vi "PlateReaderV2.vi"() -> ()   [LabVIEW 2014]
uses:
  ReadSpecifications.ctl
  TimingProfile.ctl
  PlateReaderState.ctl
  ColumnData.ctl
  RPMUpdateData.ctl
  MasterCluster.ctl
  EventHandleCommandCompletedData.ctl
  EventHandleErrorReportData.ctl
  PlateReaderGlobal.vi
  <vilib>/Instr/_visa.llb/VISA Configure Serial Port (Instr).vi
  C:/Program Files (x86)/Molecular Devices/SoftMax Pro 6.5.1 Automation SDK/SoftMaxPro.AutomationClient.dll
  Program Files (x86)/Molecular Devices/SoftMax Pro 6.5.1 Automation SDK/SoftMaxPro.AutomationClient.dll
  <vilib>/regexp/Match Regular Expression.xnode
panel:
  in  "Arduino COM Port":refnum<visa-resource-name>
  in  "Send Spoof Speed":bool
  in  "Spoof Speed (RPM)":dbl
  in  "Clear Mark Read":bool
  in  "Mark Read Stop":bool
  in  "Mark Read Start":bool
  out "Speed (RPM)":dbl
  out "Last RPM Update Time":timestamp format="%<%H:%M:%S\n%x>T"
  out "Experiment Start Time":timestamp format="%<%H:%M:%S\n%x>T"
  out "Read Count":u64
  out "Loop Iteration":i32
  out "Active Column":u64
  out "SpectraMax M5e Hardware State":string
  out "Last Column Data":T1 {"Column Mark Read Stop Time" format="%<%H:%M:%S%3u\n%x>T"; "Column Mark Read Start Time" format="%<%H:%M:%S%3u\n%x>T"; "Column Busy Stop Time" format="%<%H:%M:%S%3u\n%x>T"; "Column Busy Start Time" format="%<%H:%M:%S%3u\n%x>T"; "Column Read Start Time" format="%<%H:%M:%S%3u\n%x>T"; "Col Read Times" format="%<%H:%M:%S%3u\n%x>T"}
  out "Speed (RPM)":dbl(knob) scale=0.0..15.0
  out "Last Measured Absorbances":string[][](array[string])
  out "Position (deg)":dbl(knob) scale=0.0..360.0
  out "Message Log":string
  in  "Stop":bool
  out "LabVIEW Software State":T2
  out "SMP Return String":string
  in  "Read Specifications":T3={"Read Period (min)"=0.0, "Experiment Duration (min)"=3600.0, "Number of Columns"=12, "Apex Deviance (deg)"=90.0, "Log File Name"="Log", "Number of Wavelengths"=1, "Timing Profile"=enum."No Timing", "Column Switch Delay"=0.0, "Column Repeat Delay"=0.0, "Audible Read Delay"=0.0, "Audible Read Interval"=0.0, "SMP Protocol Path"=path "", "Upper Busy Delay Limit"=inf, "Lower Busy Delay Limit"=-inf, "Upper Busy Interval Limit"=inf, "Lower Busy Interval Limit"=-inf, "Number of Rows"=0, "Plate Reader COM Port"=""}
  in  "Start":bool
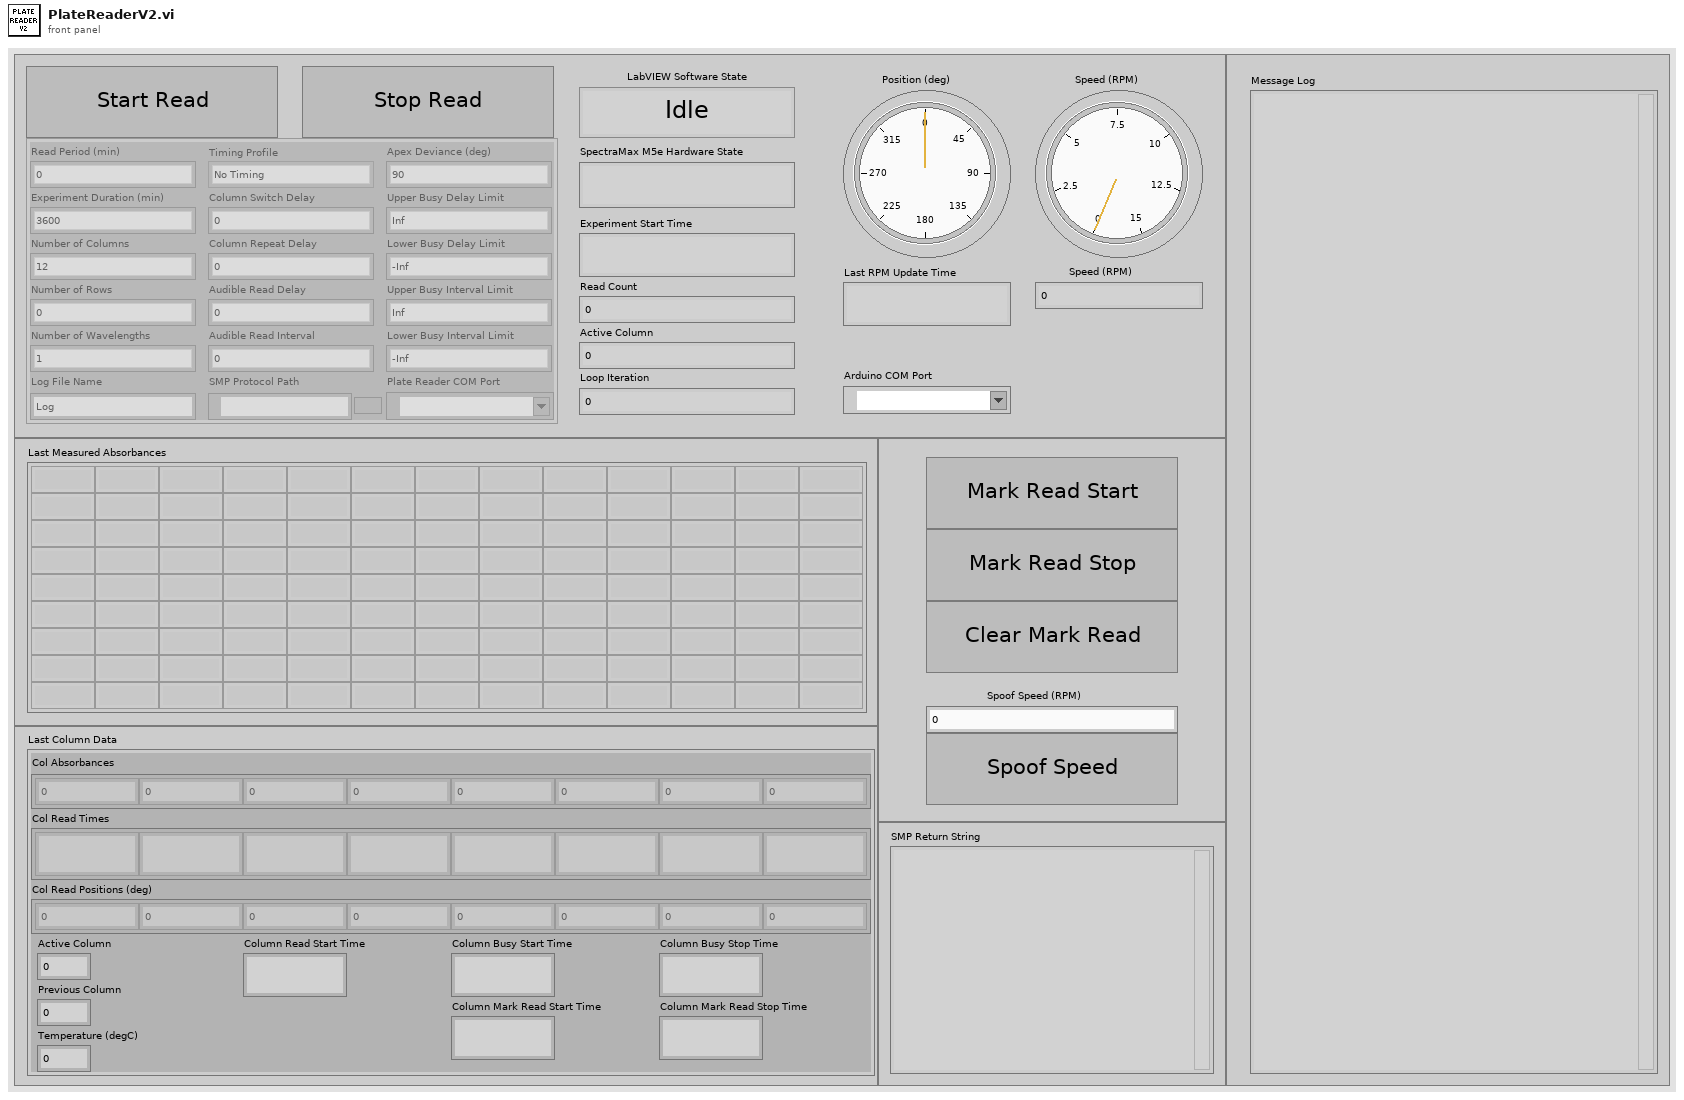
[diagram p1: front panel]
types:
  T1 = typedef "ColumnData.ctl" = cluster{"Col Absorbances":dbl[], "Col Read Times":timestamp[], "Col Read Positions (deg)":dbl[], "Temperature (degC)":dbl, "Active Column":u64, "Previous Column":u64, "Column Read Start Time":timestamp, "Column Busy Start Time":timestamp, "Column Busy Stop Time":timestamp, "Column Mark Read Start Time":timestamp, "Column Mark Read Stop Time":timestamp}
  T2 = typedef "PlateReaderState.ctl" = enum16{"Idle", "Run", "Wait", "Read", "Init", "Exit", "Stop"}
  T3 = typedef "ReadSpecifications.ctl" = cluster{"Read Period (min)":dbl, "Experiment Duration (min)":dbl, "Number of Columns":u64, "Apex Deviance (deg)":dbl, "Log File Name":string, "Number of Wavelengths":u64, "Timing Profile":T4, "Column Switch Delay":dbl, "Column Repeat Delay":dbl, "Audible Read Delay":dbl, "Audible Read Interval":dbl, "SMP Protocol Path":path, "Upper Busy Delay Limit":dbl, "Lower Busy Delay Limit":dbl, "Upper Busy Interval Limit":dbl, "Lower Busy Interval Limit":dbl, "Number of Rows":u64, "Plate Reader COM Port":refnum<visa-resource-name>}
  T4 = typedef "TimingProfile.ctl" = enum16{"No Timing", "24-Well Fluorescence", "48-Well Fluorescence", "96-Well Fluorescence", "96-Well Absorbance", "Custom Timing"}
  T5 = typedef "MasterCluster.ctl" = cluster{"Plate Reader State":T2, "SMPAutomationClientRef":refnum<k24>, "CommandCompleted Refnum":refnum<k27>, "InstrumentStatusChanged Refnum":refnum<k27>, "ErrorReport Refnum":refnum<k27>, "Read Start Time":timestamp, "Read Count":u64, "Active Column":u64, "Raw Result":string, "GetDataCopy CMD Queue ID":i32, "Error Log":string, "Column Data":T1, "Grid":dbl[][], "Column Read Start Time":timestamp, "Previous Column":u64, "Raw Log File Refnum":refnum<file>, "Read Specifications":T3, "Plate Reader Crash State":T2, "Consecutive Missed Reads":u64, "Excel File Refnum":refnum<file>}
  T6 = typedef "RPMUpdateData.ctl" = cluster{"RPM":dbl, "Last RPM Update":timestamp, "Last Position (deg)":dbl}
  T7 = typedef "EventHandleInstrumentStatusChangedData.ctl" = cluster{"Event Common Data":cluster{"Event Source":i32, "Event Type":u32, "Time Stamp":u32}, "Status":string}
  T8 = enum8{"Enabled", "Disabled", "Disabled and Grayed Out"}
  T9 = typedef "EventHandleErrorReportData.ctl" = cluster{"Event Common Data":cluster{"Event Source":i32, "Event Type":u32, "Time Stamp":u32}, "Error":string, "Command ID":i32}
  T10 = typedef "EventHandleCommandCompletedData.ctl" = cluster{"Event Common Data":cluster{"Event Source":i32, "Event Type":u32, "Time Stamp":u32}, "CommandID":i32, "DoubleResult":dbl, "IntResult":i32, "QueueEmpty":bool, "QueueID":i32, "StringResult":string}
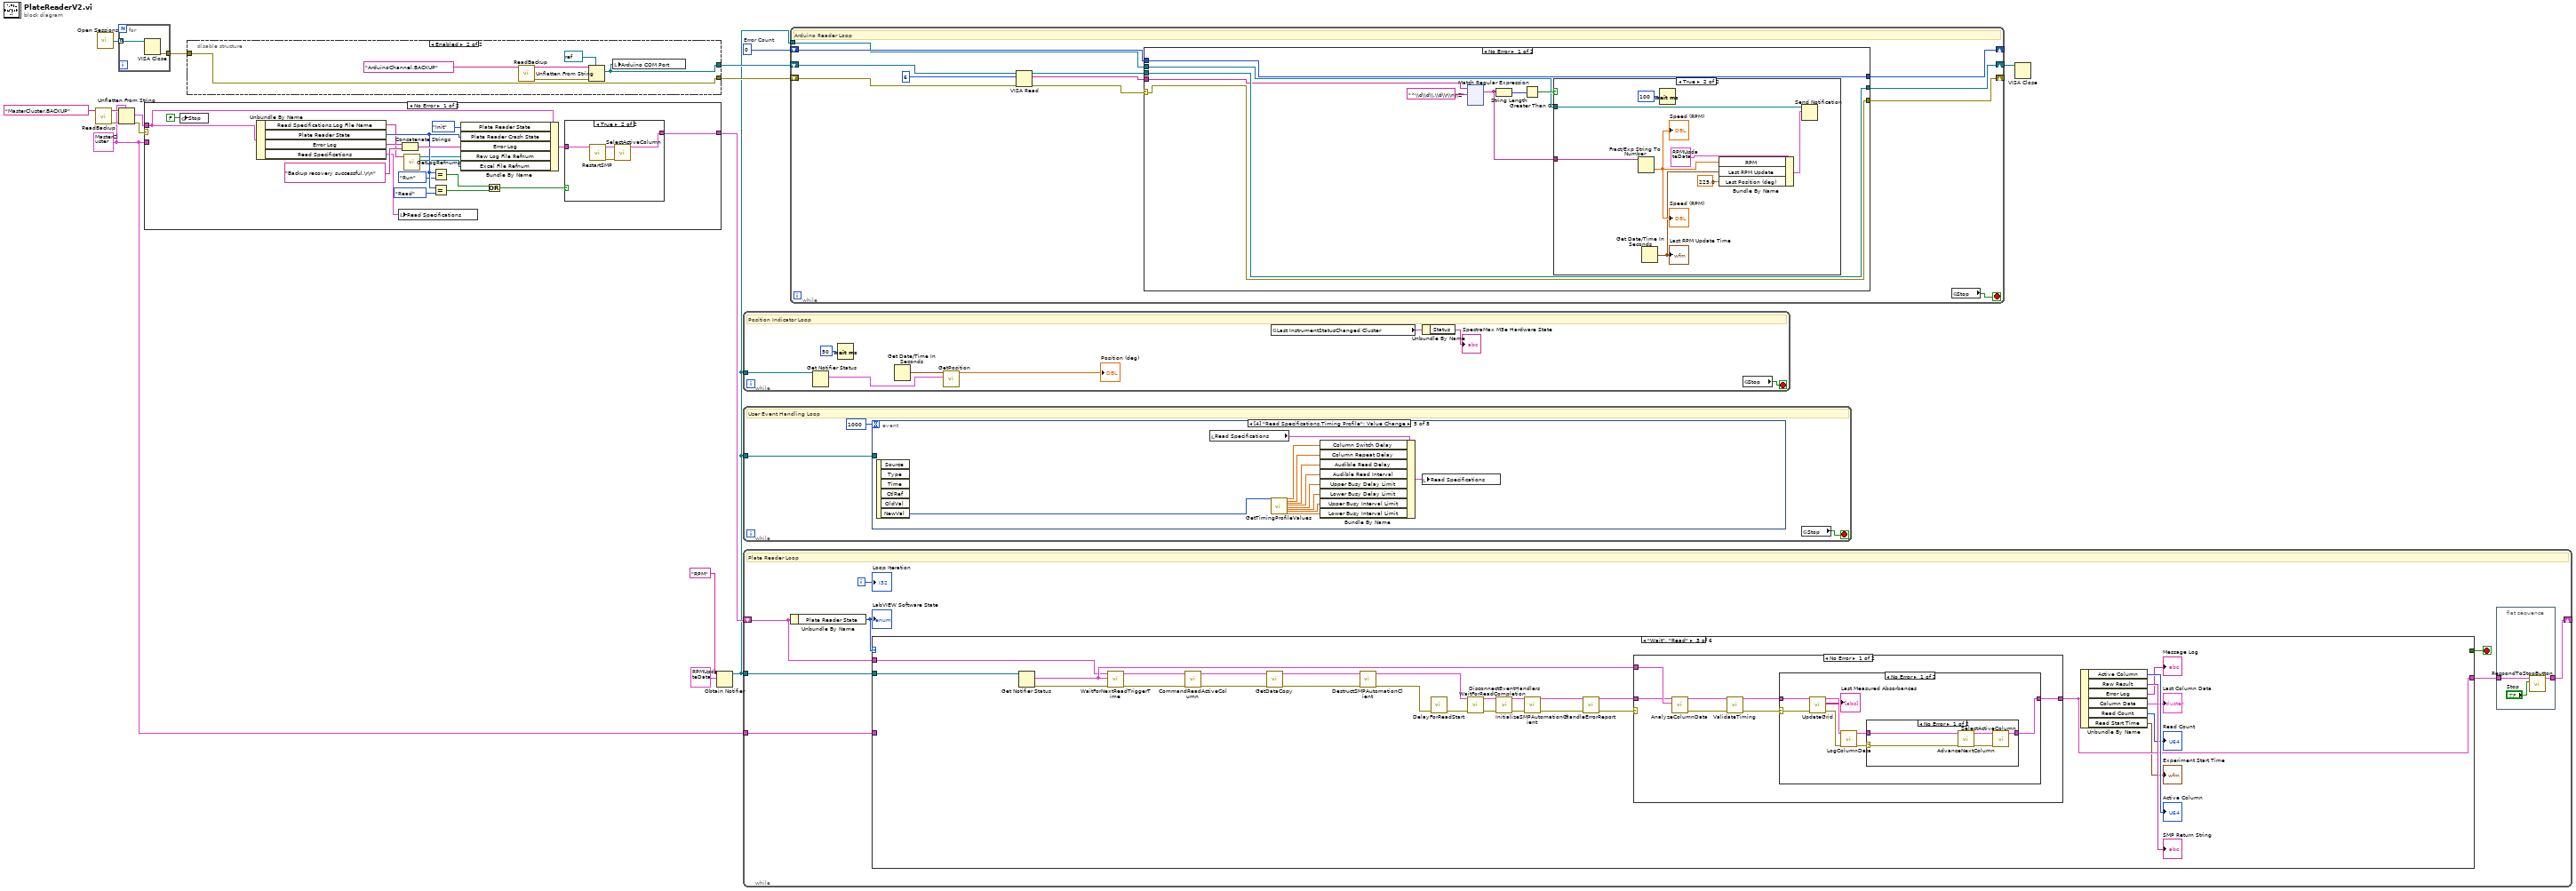
[diagram p0: block diagram]
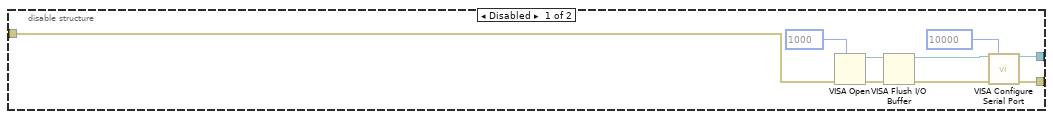
[diagram p2: hidden frame]
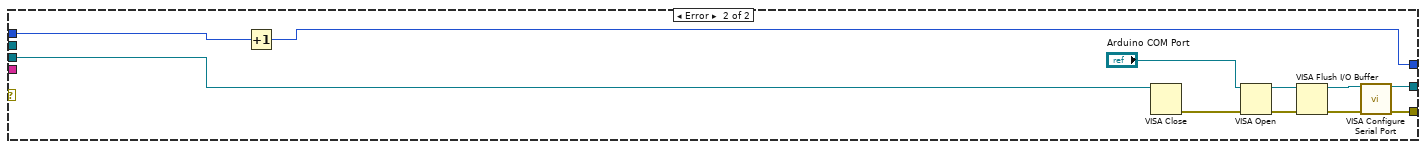
[diagram p4: hidden frame]
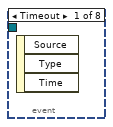
[diagram p5: hidden frame]
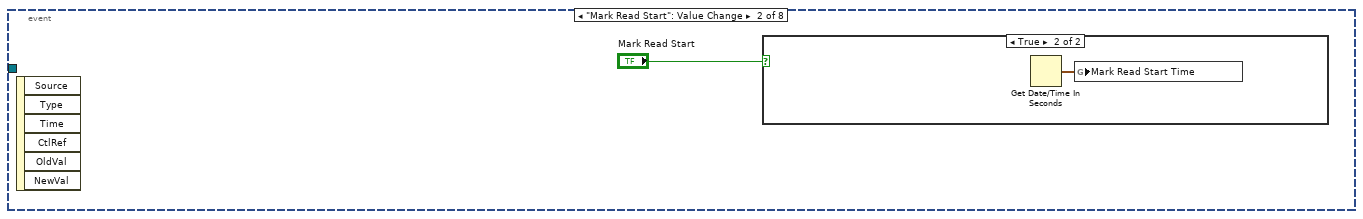
[diagram p6: hidden frame]
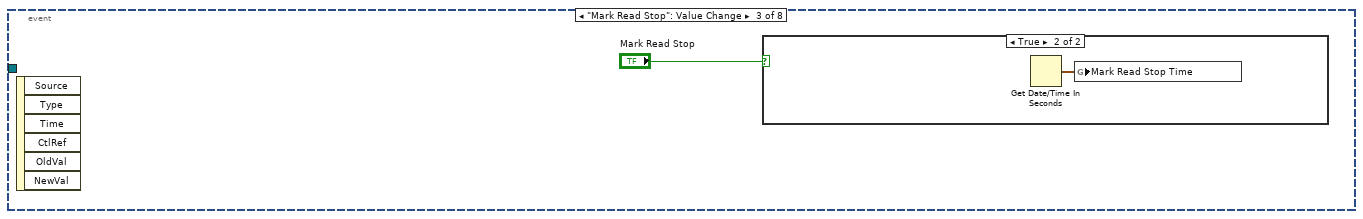
[diagram p8: hidden frame]
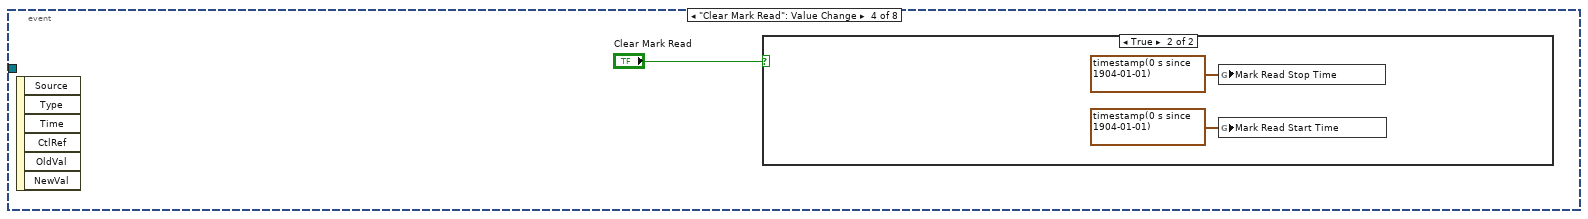
[diagram p10: hidden frame]
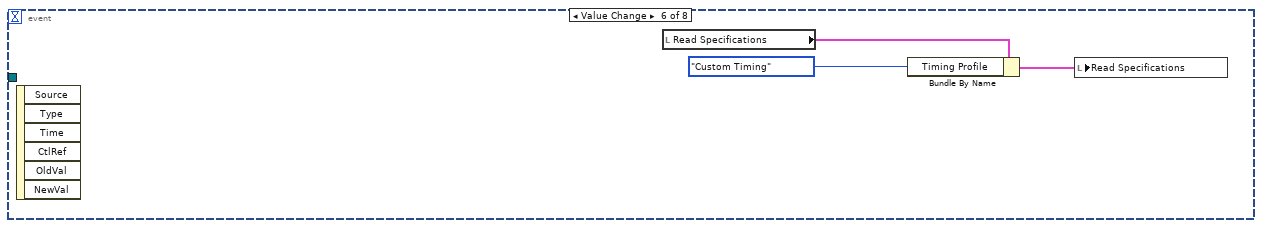
[diagram p12: hidden frame]
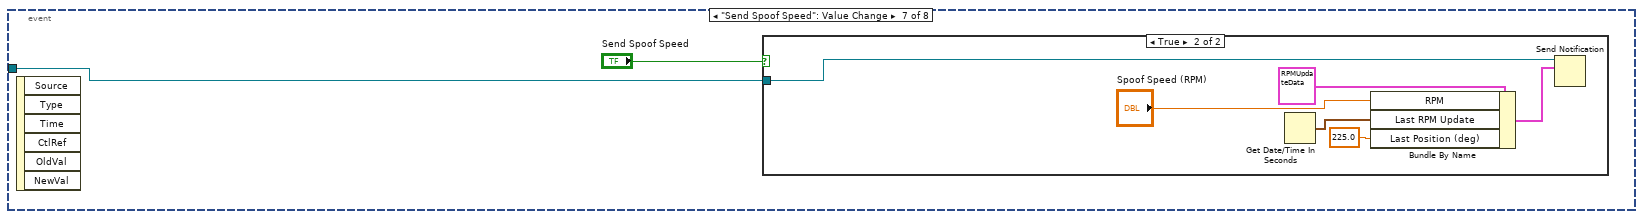
[diagram p13: hidden frame]
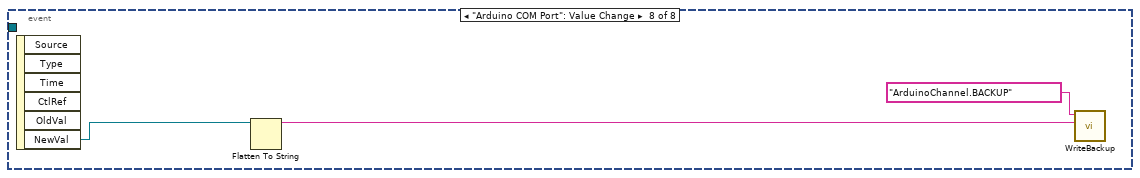
[diagram p15: hidden frame]
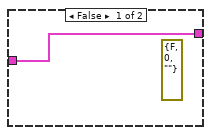
[diagram p16: hidden frame]
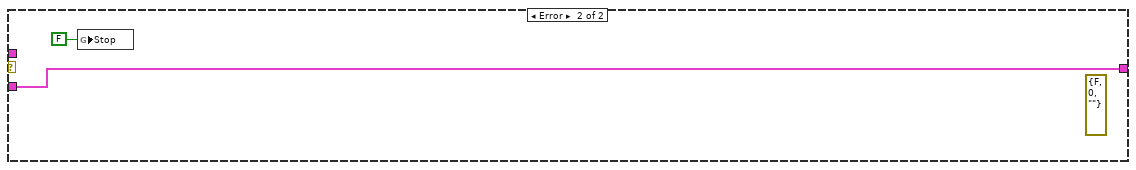
[diagram p17: hidden frame]
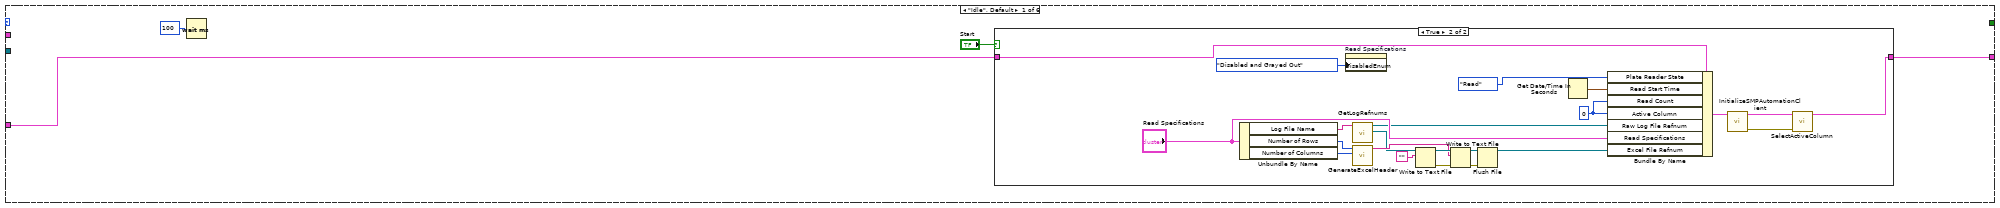
[diagram p18: hidden frame]
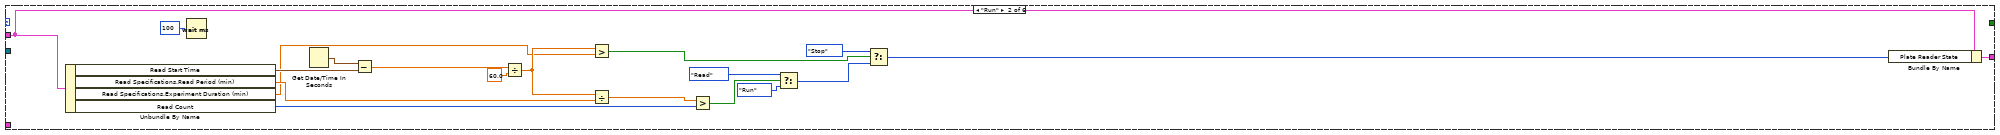
[diagram p20: hidden frame]
diagram:
  w8 = 0  # Error Count
  w1 = T5 {"Plate Reader State"=enum."Init", "SMPAutomationClientRef"=refnum, "CommandCompleted Refnum"=refnum, "InstrumentStatusChanged Refnum"=refnum, "ErrorReport Refnum"=refnum, "Read Start Time"=timestamp(0 s since 1904-01-01), "Read Count"=0, "Active Column"=0, "Raw Result"="", "GetDataCopy CMD Queue ID"=0, "Error Log"="", "Column Data"={"Col Absorbances"=[], "Col Read Times"=[], "Col Read Positions (deg)"=[], "Temperature (degC)"=0.0, "Active Column"=0, "Previous Column"=0, "Column Read Start Time"=timestamp(0 s since 1904-01-01), "Column Busy Start Time"=timestamp(0 s since 1904-01-01), "Column Busy Stop Time"=timestamp(0 s since 1904-01-01), "Column Mark Read Start Time"=timestamp(0 s since 1904-01-01), "Column Mark Read Stop Time"=timestamp(0 s since 1904-01-01)}, "Grid"=[[nan, nan, nan, nan, nan, nan, nan, nan, nan, nan, nan, nan], [nan, nan, nan, nan, nan, nan, nan, nan, nan, nan, nan, nan], [nan, nan, nan, nan, nan, nan, nan, nan, nan, nan, nan, nan], [nan, nan, nan, nan, nan, nan, nan, nan, nan, nan, nan, nan], [nan, nan, nan, nan, nan, nan, nan, nan, nan, nan, nan, nan], [nan, nan, nan, nan, nan, nan, nan, nan, nan, nan, nan, nan], [nan, nan, nan, nan, nan, nan, nan, nan, nan, nan, nan, nan], [nan, nan, nan, nan, nan, nan, nan, nan, nan, nan, nan, nan]], "Column Read Start Time"=timestamp(0 s since 1904-01-01), "Previous Column"=0, "Raw Log File Refnum"=refnum, "Read Specifications"={"Read Period (min)"=0.0, "Experiment Duration (min)"=0.0, "Number of Columns"=0, "Apex Deviance (deg)"=0.0, "Log File Name"="", "Number of Wavelengths"=0, "Timing Profile"=enum."No Timing", "Column Switch Delay"=0.0, "Column Repeat Delay"=0.0, "Audible Read Delay"=0.0, "Audible Read Interval"=0.0, "SMP Protocol Path"=path "", "Upper Busy Delay Limit"=inf, "Lower Busy Delay Limit"=-inf, "Upper Busy Interval Limit"=inf, "Lower Busy Interval Limit"=-inf, "Number of Rows"=0, "Plate Reader COM Port"=""}, "Plate Reader Crash State"=enum."Idle", "Consecutive Missed Reads"=0, "Excel File Refnum"=refnum} ("MasterCluster")
  n1 = call "ReadBackup.vi"("Backup Name"="MasterCluster.BACKUP" ("name or relative path")) -> ("error out"=w2:errorcluster, "Backup Data"=w4:string)  [unwired: 9 in]
  n2 = call <vilib>:"Open Sessions.vi"() -> ("Array of Refnums"=w10:refnum<visa-resource-name>[])  [unwired: 2 in]
  n3 = for {
    tunnel: w10 -> [w18] mode=indexing
    tunnel: [w17] -> w9
    n4 = VISA Close(VISA resource name=w18) -> (error out=w17:errorcluster)  [unwired: 1 in]
  }
  n5 = Unflatten From String(type=w1, binary string=w4, error in (no error)=w2) -> (value=w12:T5, error out=w14:errorcluster)  [unwired: 2 in, 1 out]
  n6 = case shown="No Error" w14 {
    tunnel: [w27 w43] -> w13
    tunnel: w1 -> [_ w43]
    tunnel: w12 -> [w30 _]
    frame No Error {
      n7 = global write "PlateReaderGlobal.vi" "Stop"(FALSE ("Stop")) -> ()
      n8 = Unbundle By Name(w30) -> ("Read Specifications.Log File Name"=w21:string, "Plate Reader State"=w26:T2, "Error Log"=w35:string, "Read Specifications"=w31:T3)
      n9 = local write "Read Specifications"(w31) -> ()
      n10 = Concatenate Strings(w35, "Backup recovery successful.\r\n" ("string")) -> (w33:string)
      n11 = call "GetLogRefnums.vi"("Log File Name"=w21) -> ("Excel Log Refnum"=w19:refnum<file>, "Raw Log Refnum"=w20:refnum<file>)  [unwired: 9 in]
      n12 = Equal?(x=w26, y=PlateReaderState."Run") -> (x = y?=w24:bool)
      n13 = Equal?(x=w26, y=PlateReaderState."Read") -> (x = y?=w23:bool)
      n14 = Bundle By Name(cluster=w30, "Plate Reader State"=PlateReaderState."Init", "Plate Reader Crash State"=w26, "Error Log"=w33, "Raw Log File Refnum"=w20, "Excel File Refnum"=w19) -> (w28:T5)
      n15 = Or(x=w24, y=w23) -> (x .or. y?=w22:bool)
      n16 = case shown="True" w22 {
        tunnel: w28 -> [w37 w40]
        tunnel: [w37 w41] -> w27
        frame False {
          (unwired) errorcluster {"status"=FALSE, "code"=0, "source"=""} ("Error Out")
        }
        frame True {
          n17 = call "RestartSMP.vi"("MasterCluster In"=w40) -> ("Error Out"=w38:errorcluster, "MasterCluster Out"=w39:T5)  [unwired: 9 in]
          n18 = call "SelectActiveColumn.vi"("Error In"=w38, "MasterCluster In"=w39) -> ("MasterCluster Out"=w41:T5)  [unwired: 8 in, 1 out]
        }
      }
    }
    frame Error {
      (unwired) errorcluster {"status"=FALSE, "code"=0, "source"=""} ("Error Out")
      n19 = global write "PlateReaderGlobal.vi" "Stop"(FALSE ("Stop")) -> ()
    }
  }
  n20 = disable-structure shown="Enabled" {
    disable-tunnel: w9 -> [w50 w58]
    disable-tunnel: [w47 w53] -> w7
    disable-tunnel: [w46 w58] -> w6
    frame Disabled {
      n21 = VISA Open(timeout (0)=u32 1000 ("VISA Open timeout (0)"), error in (no error)=w50) -> (VISA resource name=w51:refnum<visa-resource-name>, error out=w49:errorcluster)  [unwired: 3 in]
      n22 = VISA Flush I/O Buffer(VISA resource name=w51, error in (no error)=w49) -> (VISA resource name out=w52:refnum<visa-resource-name>, error out=w48:errorcluster)  [unwired: 1 in]
      n23 = call-poly "VISA Configure Serial Port"("VISA resource name"=w52, "timeout (10sec)"=u32 10000, "error in (no error)"=w48) -> ("VISA resource name out"=w47:refnum<visa-resource-name>, "error out"=w46:errorcluster)  [unwired: 11 in]
    }
    frame Enabled {
      n24 = call "ReadBackup.vi"("Backup Name"="ArduinoChannel.BACKUP" ("name or relative path")) -> ("error out"=w57:errorcluster, "Backup Data"=w55:string)  [unwired: 9 in]
      n25 = Unflatten From String(type=refnum<visa-resource-name> refnum ("VISA resource name out"), binary string=w55, error in (no error)=w57) -> (value=w53:refnum<visa-resource-name>)  [unwired: 2 in, 2 out]
      n26 = local write "Arduino COM Port"(w53) -> ()
    }
  }
  n27 = Obtain Notifier(name (unnamed)="RPM", notification data type=T6 {"RPM"=0.0, "Last RPM Update"=timestamp(0 s since 1904-01-01), "Last Position (deg)"=0.0} ("RPM Update Data")) -> (notifier out=w5:refnum<notifier>)  [unwired: 2 in, 2 out]
  n28 = while {
    tunnel: w5 -> [w66]
    stop <- w59 stop-if-true
    # "Position Indicator Loop"
    n29 = Get Notifier Status(notifier=w66) -> (current notification=w64:T6)  [unwired: 1 in, 4 out]
    n30 = Wait (ms)(milliseconds to wait=u32 50) -> ()  [unwired: 1 out]
    n31 = Get Date/Time In Seconds() -> (seconds since 1Jan1904=w63:timestamp)
    n32 = call "GetPosition.vi"("RPM Update Data"=w64, "Time"=w63) -> ("Position (deg)"=→"Position (deg)":dbl)  [unwired: 7 in, 2 out]
    n33 = global read "PlateReaderGlobal.vi" "Last InstrumentStatusChanged Cluster"() -> (w60:T7)
    n34 = Unbundle By Name(w60) -> ("Status"=→"SpectraMax M5e Hardware State":string)
    n35 = global read "PlateReaderGlobal.vi" "Stop"() -> (w59:bool)
  }
  n36 = while {
    tunnel: w5 -> [w67]
    stop <- w69 stop-if-true
    # "User Event Handling Loop"
    n37 = event shown="[4] \"Read Specifications.Timing Profile\": Value Change" {
      selector: _ -> [_ _ _ _ _ _ _ _]
      dyn-events: _ -> [_ _ _ _ _ _ _ _]
      timeout: 1000 -> [_ _ _ _ _ _ _ _]
      tunnel: w67 -> [_ _ _ _ _ _ w91 _]
      event Timeout {
        n38 = event-data() -> ()  [unwired: 1 in, 3 out]
      }
      event "Mark Read Start": Value Change {
        n39 = event-data() -> ()  [unwired: 1 in, 6 out]
        n40 = case shown="True" "Mark Read Start" {
          frame False {
          }
          frame True {
            n41 = Get Date/Time In Seconds() -> (seconds since 1Jan1904=w71:timestamp)
            n42 = global write "PlateReaderGlobal.vi" "Mark Read Start Time"(w71) -> ()
          }
        }
      }
      event "Mark Read Stop": Value Change {
        n43 = event-data() -> ()  [unwired: 1 in, 6 out]
        n44 = case shown="True" "Mark Read Stop" {
          frame False {
          }
          frame True {
            n45 = Get Date/Time In Seconds() -> (seconds since 1Jan1904=w73:timestamp)
            n46 = global write "PlateReaderGlobal.vi" "Mark Read Stop Time"(w73) -> ()
          }
        }
      }
      event "Clear Mark Read": Value Change {
        n47 = event-data() -> ()  [unwired: 1 in, 6 out]
        n48 = case shown="True" "Clear Mark Read" {
          frame False {
          }
          frame True {
            n49 = global write "PlateReaderGlobal.vi" "Mark Read Stop Time"(timestamp(0 s since 1904-01-01) ("Mark Read Stop Time")) -> ()
            n50 = global write "PlateReaderGlobal.vi" "Mark Read Start Time"(timestamp(0 s since 1904-01-01) ("Mark Read Start Time")) -> ()
          }
        }
      }
      event Value Change {
        n51 = event-data() -> ("NewVal"=w86:T4)  [unwired: 1 in, 5 out]
        n52 = local read "Read Specifications"() -> (w87:T3)
        n53 = call "GetTimingProfileValues.vi"("Timing Profile"=w86) -> ("Column Switch Command Delay"=w84:dbl, "Column Repeat Command Delay"=w83:dbl, "Audible Read Delay"=w82:dbl, "Audible Read Interval"=w81:dbl, "Upper Busy Delay Limit"=w80:dbl, "Lower Busy Delay Limit"=w79:dbl, "Upper Busy Interval Limit"=w78:dbl, "Lower Busy Interval Limit"=w77:dbl)  [unwired: 19 in]
        n54 = Bundle By Name(cluster=w87, "Column Switch Delay"=w84, "Column Repeat Delay"=w83, "Audible Read Delay"=w82, "Audible Read Interval"=w81, "Upper Busy Delay Limit"=w80, "Lower Busy Delay Limit"=w79, "Upper Busy Interval Limit"=w78, "Lower Busy Interval Limit"=w77) -> (w85:T3)
        n55 = local write "Read Specifications"(w85) -> ()
      }
      event Value Change {
        n56 = event-data() -> ()  [unwired: 1 in, 6 out]
        n57 = local read "Read Specifications"() -> (w90:T3)
        n58 = Bundle By Name(cluster=w90, "Timing Profile"=TimingProfile."Custom Timing") -> (w88:T3)
        n59 = local write "Read Specifications"(w88) -> ()
      }
      event "Send Spoof Speed": Value Change {
        n60 = event-data() -> ()  [unwired: 1 in, 6 out]
        n61 = case shown="True" "Send Spoof Speed" {
          tunnel: w91 -> [_ w93]
          frame False {
          }
          frame True {
            n62 = Get Date/Time In Seconds() -> (seconds since 1Jan1904=w97:timestamp)
            n63 = Bundle By Name(cluster=T6 {"RPM"=0.0, "Last RPM Update"=timestamp(0 s since 1904-01-01), "Last Position (deg)"=0.0} ("RPM Update Data"), "RPM"="Spoof Speed (RPM)", "Last RPM Update"=w97, "Last Position (deg)"=225.0) -> (w95:T6)
            n64 = Send Notification(notification=w95, notifier=w93) -> ()  [unwired: 1 in, 2 out]
          }
        }
      }
      event "Arduino COM Port": Value Change {
        n65 = event-data() -> ("NewVal"=w99:refnum<visa-resource-name>)  [unwired: 1 in, 5 out]
        n66 = Flatten To String(anything=w99) -> (data string=w100:string)  [unwired: 3 in, 2 out]
        n67 = call "WriteBackup.vi"("Backup Data"=w100, "Backup Name"="ArduinoChannel.BACKUP" ("name or relative path")) -> ()  [unwired: 10 in]
      }
    }
    n68 = global read "PlateReaderGlobal.vi" "Stop"() -> (w69:bool)
  }
  n69 = while {
    shift-right: [w103] -> _
    shift-left: w13 -> [w109]
    tunnel: w5 -> [w107]
    tunnel: w1 -> [w102]
    i -> [w106]
    stop <- w108 stop-if-true
    # "Plate Reader Loop"
    n70 = Unbundle By Name(w109) -> ("Plate Reader State"=w105:T2)
    "LabVIEW Software State" <- w105
    n71 = case shown="\"Wait\", \"Read\"" w105 {
      tunnel: w109 -> [_ w142 w172 w216 w229 w239]
      tunnel: [w114 w140 w177 w217 w229 w247] -> w104
      tunnel: [_ _ _ _ w235 _] -> w108
      tunnel: w107 -> [_ _ w186 _ _ _]
      tunnel: w102 -> [w113 _ _ _ w232 w238]
      frame "Idle", Default {
        n72 = Wait (ms)(milliseconds to wait=u32 100) -> ()  [unwired: 1 out]
        n73 = case shown="True" "Start" {
          tunnel: [w117 w133] -> w114
          tunnel: w113 -> [w117 w139]
          frame False {
          }
          frame True {
            w136 = u64 0 ("Read Count")
            n74 = Unbundle By Name("Read Specifications") -> ("Log File Name"=w120:string, "Number of Rows"=w124:u64, "Number of Columns"=w121:u64)
            n75 = property on="Read Specifications" class="Clust (strict)"("DisabledEnum"=T8."Disabled and Grayed Out" ("Disabled")) -> ()  [unwired: 2 in, 2 out]
            n76 = call "GetLogRefnums.vi"("Log File Name"=w120) -> ("Excel Log Refnum"=w118:refnum<file>, "Raw Log Refnum"=w119:refnum<file>)  [unwired: 9 in]
            n77 = call "GenerateExcelHeader.vi"("Number of Columns"=w121, "Number of Rows"=w124) -> ("Excel Header"=w123:string)  [unwired: 9 in]
            n78 = Write to Text File(file (use dialog)=w118, text="") -> (refnum out=w128:refnum<file>, error out=w127:errorcluster)  [unwired: 2 in, 1 out]
            n79 = Write to Text File(file (use dialog)=w128, text=w123, error in=w127) -> (refnum out=w126:refnum<file>, error out=w125:errorcluster)  [unwired: 1 in, 1 out]
            n80 = Flush File(refnum=w126, error in=w125) -> (refnum out=w122:refnum<file>)  [unwired: 1 out]
            n81 = Get Date/Time In Seconds() -> (seconds since 1Jan1904=w137:timestamp)
            n82 = Bundle By Name(cluster=w139, "Plate Reader State"=PlateReaderState."Read", "Read Start Time"=w137, "Read Count"=w136, "Active Column"=w136, "Raw Log File Refnum"=w119, "Read Specifications"="Read Specifications", "Excel File Refnum"=w122) -> (w132:T5)
            n83 = call "InitializeSMPAutomationClient.vi"("MasterCluster In"=w132) -> ("Error Out"=w130:errorcluster, "MasterCluster Out"=w131:T5)  [unwired: 9 in]
            n84 = call "SelectActiveColumn.vi"("Error In"=w130, "MasterCluster In"=w131) -> ("MasterCluster Out"=w133:T5)  [unwired: 8 in, 1 out]
          }
        }
      }
      frame "Run" {
        n85 = Unbundle By Name(w142) -> ("Read Start Time"=w146:timestamp, "Read Specifications.Read Period (min)"=w145:dbl, "Read Specifications.Experiment Duration (min)"=w144:dbl, "Read Count"=w143:u64)
        n86 = Wait (ms)(milliseconds to wait=u32 100) -> ()  [unwired: 1 out]
        n87 = Get Date/Time In Seconds() -> (seconds since 1Jan1904=w157:timestamp)
        n88 = Subtract(x=w157, y=w146) -> (x-y=w156:dbl)
        n89 = Divide(x=w156, y=60.0) -> (x/y=w152:dbl)
        n90 = Greater?(x=w152, y=w144) -> (0:w154:bool)
        n91 = Divide(x=w152, y=w145) -> (x/y=w151:dbl)
        n92 = Greater?(x=w151, y=w143) -> (0:w149:bool)
        n93 = Select(t=PlateReaderState."Read" ("Plate Reader State"), s=w149, f=PlateReaderState."Run" ("Plate Reader State")) -> (s? t:f=w150:T2)
        n94 = Select(t=PlateReaderState."Stop" ("Plate Reader State"), s=w154, f=w150) -> (s? t:f=w141:T2)
        n95 = Bundle By Name(cluster=w142, "Plate Reader State"=w141) -> (w140:T5)
      }
      frame "Wait", "Read" {
        n96 = Get Notifier Status(notifier=w186) -> (current notification=w173:T6, error out=w185:errorcluster)  [unwired: 1 in, 3 out]
        n97 = call "WaitForNextReadTriggerTime.vi"("Error In"=w185, "RPM Update Data"=w173, "MasterCluster In"=w172) -> ("Error Out"=w168:errorcluster, "MasterCluster Out"=w169:T5)  [unwired: 6 in, 1 out]
        n98 = call "CommandReadActiveColumn.vi"("Error In"=w168, "MasterCluster In"=w169) -> ("Error Out"=w159:errorcluster, "MasterCluster Out"=w162:T5)  [unwired: 7 in, 1 out]
        n99 = call "GetDataCopy.vi"("Error In"=w159, "MasterCluster In"=w162) -> ("Error Out"=w160:errorcluster, "MasterCluster Out"=w161:T5)  [unwired: 8 in]
        n100 = call "DestructSMPAutomationClient.vi"("Error In"=w160, "MasterCluster In"=w161) -> ("Error Out"=w163:errorcluster, "MasterCluster Out"=w170:T5)  [unwired: 8 in]
        n101 = call "DelayForReadStart.vi"("Error In"=w163) -> ("Error Out"=w171:errorcluster)  [unwired: 10 in]
        n102 = call "WaitForReadCompletion.vi"("Error In"=w171, "MasterCluster In"=w170) -> ("Error Out"=w184:errorcluster, "MasterCluster Out"=w183:T5)  [unwired: 7 in, 1 out]
        n103 = call "DisconnectEventHandlers.vi"("Error In"=w184, "MasterCluster In"=w183) -> ("Error Out"=w166:errorcluster, "MasterCluster Out"=w167:T5)  [unwired: 8 in]
        n104 = call "InitializeSMPAutomationClient.vi"("Error In"=w166, "MasterCluster In"=w167) -> ("Error Out"=w164:errorcluster, "MasterCluster Out"=w165:T5)  [unwired: 8 in]
        n105 = call "HandleErrorReport.vi"("Error In"=w164, "MasterCluster In"=w165) -> ("Error Out"=w179:errorcluster, "MasterCluster Out"=w178:T5)  [unwired: 8 in]
        n106 = case shown="No Error" w179 {
          selector: w179 -> [_ w215]
          tunnel: w178 -> [w192 w214]
          tunnel: [w191 w213] -> w177
          tunnel: w173 -> [w193 _]
          frame No Error {
            n107 = call "AnalyzeColumnData.vi"("RPM Update Data"=w193, "MasterCluster In"=w192) -> ("Error Out"=w187:errorcluster, "MasterCluster Out"=w190:T5)  [unwired: 8 in]
            n108 = call "ValidateTiming.vi"("Error In"=w187, "MasterCluster In"=w190) -> ("Error Out"=w188:errorcluster, "MasterCluster Out"=w189:T5)  [unwired: 8 in]
            n109 = case shown="No Error" w188 {
              selector: w188 -> [w195 w211]
              tunnel: [w200 w210] -> w191
              tunnel: w189 -> [w199 w212]
              frame No Error {
                n110 = call "UpdateGrid.vi"("Error In"=w195, "MasterCluster In"=w199) -> ("Error Out"=w197:errorcluster, "ASCII Grid"=→"Last Measured Absorbances":string[][], "MasterCluster Out"=w198:T5)  [unwired: 7 in]
                n111 = call "LogColumnData.vi"("Error In"=w197, "MasterCluster In"=w198) -> ("Error Out"=w194:errorcluster, "MasterCluster Out"=w201:T5)  [unwired: 8 in]
                n112 = case shown="No Error" w194 {
                  selector: w194 -> [w205 w207]
                  tunnel: w201 -> [w206 w209]
                  tunnel: [w202 w208] -> w200
                  frame No Error {
                    n113 = call "AdvanceNextColumn.vi"("Error In"=w205, "MasterCluster In"=w206) -> ("Error Out"=w203:errorcluster, "MasterCluster Out"=w204:T5)  [unwired: 8 in]
                    n114 = call "SelectActiveColumn.vi"("Error In"=w203, "MasterCluster In"=w204) -> ("MasterCluster Out"=w202:T5)  [unwired: 8 in, 1 out]
                  }
                  frame Error {
                    n115 = call "HandleLabVIEWErrors.vi"("Error In"=w207, "MasterCluster In"=w209) -> ("MasterCluster Out"=w208:T5)  [unwired: 9 in]
                  }
                }
              }
              frame Error {
                n116 = call "HandleLabVIEWErrors.vi"("Error In"=w211, "MasterCluster In"=w212) -> ("MasterCluster Out"=w210:T5)  [unwired: 9 in]
              }
            }
          }
          frame Error {
            n117 = call "HandleLabVIEWErrors.vi"("Error In"=w215, "MasterCluster In"=w214) -> ("MasterCluster Out"=w213:T5)  [unwired: 9 in]
          }
        }
        n118 = Unbundle By Name(w177) -> ("Active Column"=→"Active Column":u64, "Raw Result"=→"SMP Return String":string, "Error Log"=→"Message Log":string, "Column Data"=→"Last Column Data":T1, "Read Count"=→"Read Count":u64, "Read Start Time"=→"Experiment Start Time":timestamp)
      }
      frame "Init" {
        n119 = property on="Position (deg)" class="Knob (strict)"("Scale.SclPosRange"=6.283185307179586, "Scale.SclPosStart"=1.5707963267948966) -> ()  [unwired: 2 in, 2 out]
        n120 = property on="Read Specifications" class="Clust (strict)"("DisabledEnum"=T8."Enabled" ("Disabled")) -> ()  [unwired: 2 in, 2 out]
        n121 = Obtain Queue(name (unnamed)="ErrorReportQueue", element data type=T9 {"Event Common Data"={"Event Source"=0, "Event Type"=0, "Time Stamp"=0}, "Error"="", "Command ID"=0} ("ErrorReport Data")) -> (queue out=w222:refnum<queue>)  [unwired: 3 in, 2 out]
        n122 = global write "PlateReaderGlobal.vi" "ErrorReportQueue"(w222) -> ()
        n123 = Obtain Queue(name (unnamed)="CommandCompleteQueue", element data type=T10 {"Event Common Data"={"Event Source"=0, "Event Type"=0, "Time Stamp"=0}, "CommandID"=0, "DoubleResult"=0.0, "IntResult"=0, "QueueEmpty"=FALSE, "QueueID"=0, "StringResult"=""} ("Event Data Cluster")) -> (queue out=w225:refnum<queue>)  [unwired: 3 in, 2 out]
        n124 = global write "PlateReaderGlobal.vi" "CommandCompleteQueue"(w225) -> ()
        n125 = Unbundle By Name(w216) -> ("Plate Reader Crash State"=w218:T2)
        n126 = Bundle By Name(cluster=w216, "Plate Reader State"=w218) -> (w217:T5)
      }
      frame "Exit" {
        w228 = PlateReaderState."Idle" ("Plate Reader Crash State")
        w235 = TRUE
        n127 = Unbundle By Name(w229) -> ("Read Specifications"=w231:T3)
        n128 = Bundle By Name(cluster=w232, "Read Specifications"=w231, "Plate Reader Crash State"=w228, "Plate Reader State"=w228) -> (w230:T5)
        n129 = Flatten To String(anything=w230) -> (data string=w233:string)  [unwired: 3 in, 2 out]
        n130 = call "WriteBackup.vi"("Backup Data"=w233, "Backup Name"="MasterCluster.BACKUP" ("name or relative path")) -> ()  [unwired: 10 in]
        n131 = global write "PlateReaderGlobal.vi" "Stop"(w235) -> ()
      }
      frame "Stop" {
        w237 = PlateReaderState."Idle" ("Plate Reader Crash State")
        n132 = Unbundle By Name(w239) -> ("Raw Log File Refnum"=w249:refnum<file>, "Excel File Refnum"=w243:refnum<file>, "Read Specifications"=w236:T3)
        n133 = Close File(refnum=w249) -> ()  [unwired: 1 in, 2 out]
        n134 = Close File(refnum=w243) -> ()  [unwired: 1 in, 2 out]
        n135 = property on="Read Specifications" class="Clust (strict)"("DisabledEnum"=T8."Enabled" ("Disabled")) -> ()  [unwired: 2 in, 2 out]
        n136 = Bundle By Name(cluster=w238, "Read Specifications"=w236, "Plate Reader Crash State"=w237, "Plate Reader State"=w237) -> (w240:T5)
        n137 = Flatten To String(anything=w240) -> (data string=w241:string)  [unwired: 3 in, 2 out]
        n138 = call "WriteBackup.vi"("Backup Data"=w241, "Backup Name"="MasterCluster.BACKUP" ("name or relative path")) -> ()  [unwired: 10 in]
        n139 = call "DestructSMPAutomationClient.vi"("MasterCluster In"=w239) -> ("MasterCluster Out"=w245:T5)  [unwired: 9 in, 1 out]
        n140 = call "DisconnectEventHandlers.vi"("MasterCluster In"=w245) -> ("MasterCluster Out"=w244:T5)  [unwired: 9 in, 1 out]
        n141 = Bundle By Name(cluster=w244, "Plate Reader State"=PlateReaderState."Idle") -> (w247:T5)
      }
    }
    n142 = flat-sequence {
      tunnel: [w112] -> w103
      tunnel: w104 -> [w111]
      frame #0 {
        n143 = call "RespondToStopButton.vi"("Stop"="Stop", "Master Cluster In"=w111) -> ("Master Cluster Out"=w112:T5)  [unwired: 9 in]
      }
    }
    "Loop Iteration" <- w106
  }
  n144 = while {
    shift-right: [w256] -> w11
    shift-left: w7 -> [w261]
    shift-right: [w258] -> _
    shift-left: w8 -> [w259]
    shift-right: [w253] -> _
    shift-left: w6 -> [w254]
    tunnel: w5 -> [w251]
    stop <- w252 stop-if-true
    # "Arduino Reader Loop"
    n145 = VISA Read(VISA resource name=w261, byte count=u32 6, error in (no error)=w254) -> (VISA resource name out=w257:refnum<visa-resource-name>, read buffer=w255:string, error out=w250:errorcluster)  [unwired: 1 out]
    n146 = case shown="No Error" w250 {
      selector: w250 -> [w262 _]
      tunnel: w259 -> [w270 w403]
      tunnel: [w270 w402] -> w258
      tunnel: w257 -> [w269 w397]
      tunnel: [w269 w398] -> w256
      tunnel: w255 -> [w264 _]
      tunnel: [w262 w394] -> w253
      tunnel: w251 -> [w263 _]
      frame No Error {
        n147 = xnode "Match Regular Expression"("input string"=w264, "regular expression"="^\\d\\d\\.\\d\\r\\n\\Z") -> ("whole match"=w267:string)  [unwired: 4 in, 4 out]
        n148 = String Length(string=w267) -> (length=w265:i32)
        n149 = Greater Than 0?(x=w265) -> (x > 0?=w266:bool)
        n150 = case shown="True" w266 {
          tunnel: w267 -> [_ w278]
          tunnel: w263 -> [_ w273]
          frame False {
          }
          frame True {
            n151 = Fract/Exp String To Number(string=w278) -> (number=w275:dbl)  [unwired: 3 in, 1 out]
            "Speed (RPM)" <- w275
            "Speed (RPM)" <- w275
            n152 = Get Date/Time In Seconds() -> (seconds since 1Jan1904=w274:timestamp)
            "Last RPM Update Time" <- w274
            n153 = Wait (ms)(milliseconds to wait=u32 100) -> ()  [unwired: 1 out]
            n154 = Bundle By Name(cluster=T6 {"RPM"=0.0, "Last RPM Update"=timestamp(0 s since 1904-01-01), "Last Position (deg)"=0.0} ("RPM Update Data"), "RPM"=w275, "Last RPM Update"=w274, "Last Position (deg)"=225.0) -> (w272:T6)
            n155 = Send Notification(notification=w272, notifier=w273) -> ()  [unwired: 1 in, 2 out]
          }
        }
      }
      frame Error {
        n156 = Increment(x=w403) -> (x+1=w402:i32)
        n157 = VISA Close(VISA resource name=w397) -> (error out=w401:errorcluster)  [unwired: 1 in]
        n158 = VISA Open(error in (no error)=w401, VISA resource name="Arduino COM Port") -> (VISA resource name=w400:refnum<visa-resource-name>, error out=w396:errorcluster)  [unwired: 3 in]
        n159 = VISA Flush I/O Buffer(VISA resource name=w400, error in (no error)=w396) -> (VISA resource name out=w399:refnum<visa-resource-name>, error out=w395:errorcluster)  [unwired: 1 in]
        n160 = call-poly "VISA Configure Serial Port"("VISA resource name"=w399, "error in (no error)"=w395) -> ("VISA resource name out"=w398:refnum<visa-resource-name>, "error out"=w394:errorcluster)  [unwired: 12 in]
      }
    }
    n161 = global read "PlateReaderGlobal.vi" "Stop"() -> (w252:bool)
  }
  n162 = VISA Close(VISA resource name=w11) -> ()  [unwired: 1 in, 1 out]
